vi "Stacking Test.vi"(11 "Pilot-CoPilot Gamepad Controls":T1) -> ()   [LabVIEW 2014]
uses:
  Subsystems VIs/Robot Control Outputs 2015.ctl
  <vilib>/Rock Robotics/WPI/Solenoid/WPI_SolenoidValue.ctl
  <vilib>/Rock Robotics/Network Tables/SD Write Boolean Array.vi
  Global Variables/Refnum Names.vi
  Global Variables/Sensor Data (Edited).vi
  <vilib>/Rock Robotics/Network Tables/SD Write Numeric Array.vi
  <vilib>/Rock Robotics/Network Tables/SD Write Boolean.vi
  <vilib>/Rock Robotics/WPI/Solenoid/WPI_SolenoidSetEnum.vi
panel:
  out "Motor Output":dbl
  # "CB = control board"
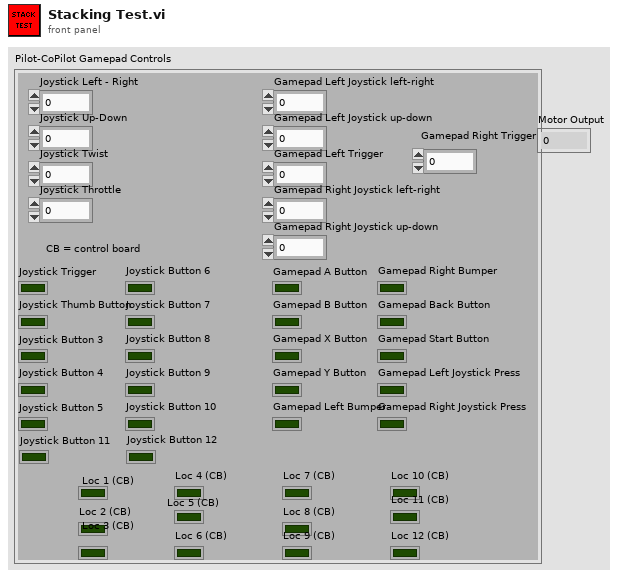
[diagram p1: front panel]
types:
  T1 = typedef "Robot Control Outputs 2015.ctl" = cluster{"Gamepad Left Joystick left-right":dbl, "Gamepad Left Joystick up-down":dbl, "Gamepad A Button":bool, "Gamepad B Button":bool, "Gamepad X Button":bool, "Gamepad Y Button":bool, "Gamepad Left Bumper":bool, "Gamepad Right Bumper":bool, "Gamepad Back Button":bool, "Gamepad Start Button":bool, "Gamepad Left Joystick Press":bool, "Gamepad Right Joystick Press":bool, "Joystick Trigger":bool, "Joystick Thumb Button":bool, "Joystick Button 3":bool, "Joystick Button 4":bool, "Joystick Button 5":bool, "Joystick Button 6":bool, "Joystick Button 7":bool, "Joystick Button 8":bool, "Joystick Button 9":bool, "Joystick Button 10":bool, "Gamepad Left Trigger":dbl, "Gamepad Right Joystick left-right":dbl, "Gamepad Right Joystick up-down":dbl, "Joystick Left - Right":dbl, "Joystick Up-Down":dbl, "Joystick Twist":dbl, "Joystick Throttle":dbl, "Loc 1 (CB)":bool, "Loc 4 (CB)":bool, "Gamepad Right Trigger":dbl, "Loc 2 (CB)":bool, "Loc 3 (CB)":bool, "Loc 5 (CB)":bool, "Loc 6 (CB)":bool, "Loc 7 (CB)":bool, "Loc 10 (CB)":bool, "Loc 8 (CB)":bool, "Loc 9 (CB)":bool, "Loc 11 (CB)":bool, "Loc 12 (CB)":bool, "Joystick Button 11":bool, "Joystick Button 12":bool}
  T2 = typedef "WPI_SolenoidValue.ctl" = enum16{"Off", "On", "Forward", "Reverse"}
  T3 = typedef "WPI_SolenoidDevRef.ctl" = cluster{"DevStatus":errorcluster, "Pneumatics Control Module":u8, "Forward Solenoid Channel":T4, "Reverse Solenoid Channel":T4}
  T4 = typedef "WPI_SolenoidChannel.ctl" = enum8{"Solenoid 0", "Solenoid 1", "Solenoid 2", "Solenoid 3", "Solenoid 4", "Solenoid 5", "Solenoid 6", "Solenoid 7", "Invalid"}
  T5 = typedef "WPI_MotorControlDeviceRef.ctl" = cluster{"DeviceStatus":errorcluster, "Type":T6, "PWM":cluster{"Controller":T7, "PWM Channel":T8, "DeadBand":T9}, "CAN":cluster{"Device Number":u8, "Control Mode":T10, "Semaphore":T11, "Max Vout":dbl, "TalonSRX Control Mode":T12}, "Invert":bool, "TransformRef":T13, "InvTransformRef":T13}
  T6 = typedef "WPI_MotorControlType.ctl" = enum16{"PWM", "CAN", "CANTalonSRX"}
  T7 = typedef "FPGA_TypedefDigitalModule.ctl" = enum16{"Controller 1"}
  T8 = typedef "FPGA_DIOPWMChannel.ctl" = enum8{"PWM 0", "PWM 1", "PWM 2", "PWM 3", "PWM 4", "PWM 5", "PWM 6", "PWM 7", "PWM 8", "PWM 9", "PWM MXP 0", "PWM MXP 1", "PWM MXP 2", "PWM MXP 3", "PWM MXP 4", "PWM MXP 5", "PWM MXP 6", "PWM MXP 7", "PWM MXP 8", "PWM MXP 9", "Invalid"}
  T9 = typedef "WPI_PWMDeadband.ctl" = cluster{"Name":string, "maxPositivePwm":i32, "minPositivePwm":i32, "centerPwm":i32, "maxNegativePwm":i32, "minNegativePwm":i32, "angularRange":u16}
  T10 = typedef "WPI_CANJaguar_ControlMode.ctl" = enum8{"Percent VBus", "Current", "Speed", "Position", "Voltage"}
  T11 = typedef "Semaphore RefNum" = refnum<k1>
  T12 = typedef "WPI_CANTalonSRX_APIControlMode.ctl" = enum8{"Percent VBus", "Speed", "Position", "Slave", "Unchanged / Invalid"}
  T13 = typedef "WPI_PWMTransform_ConPane.ctl" = refnum<vi>
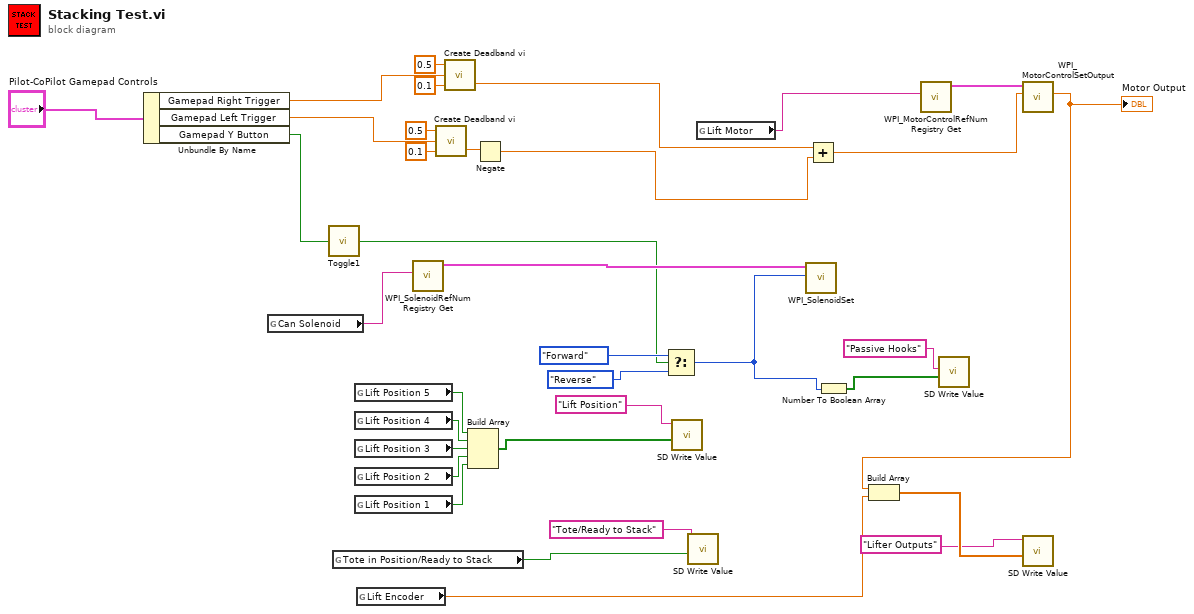
[diagram p0: block diagram]
diagram:
  n1 = Unbundle By Name("Pilot-CoPilot Gamepad Controls") -> ("Gamepad Right Trigger"=w9:dbl, "Gamepad Left Trigger"=w4:dbl, "Gamepad Y Button"=w34:bool)
  n2 = global read "Refnum Names.vi" "Can Solenoid"() -> (w13:string)
  n3 = call "Toggle1.vi"("Boolean"=w34) -> ("Driver Switch 2"=w14:bool)
  n4 = global read "Sensor Data (Edited).vi" "Tote in Position/Ready to Stack"() -> (w19:bool)
  n5 = global read "Sensor Data (Edited).vi" "Lift Position 5"() -> (w33:bool)
  n6 = global read "Sensor Data (Edited).vi" "Lift Position 4"() -> (w32:bool)
  n7 = global read "Sensor Data (Edited).vi" "Lift Position 3"() -> (w31:bool)
  n8 = global read "Sensor Data (Edited).vi" "Lift Position 2"() -> (w30:bool)
  n9 = global read "Sensor Data (Edited).vi" "Lift Position 1"() -> (w29:bool)
  n10 = global read "Sensor Data (Edited).vi" "Lift Encoder"() -> (w24:dbl)
  n11 = call <vilib>:"WPI_SolenoidRefNum Registry Get.vi"("refnum name"=w13) -> ("SolenoidDevRef"=w17:T3)  [unwired: 9 in, 1 out]
  n12 = call "Create Deadband vi.vi"("Input Deadband"=0.1, "Input"=w4, "Output Upper Limit"=0.5) -> ("Output"=w3:dbl)  [unwired: 1 in]
  n13 = call "Create Deadband vi.vi"("Input Deadband"=0.1, "Input"=w9, "Output Upper Limit"=0.5) -> ("Output"=w1:dbl)  [unwired: 1 in]
  n14 = Build Array(w33, w32, w31, w30, w29) -> (w28:bool[])
  n15 = Negate(x=w3) -> (-x=w2:dbl)
  n16 = Select(t=WPI_SolenoidValue."Forward" ("Value"), s=w14, f=WPI_SolenoidValue."Reverse" ("Value")) -> (s? t:f=w12:T2)
  n17 = call-poly <vilib>:"SD Write Value.vi"("Boolean Array"=w28, "Name"="Lift Position") -> ()  [unwired: 8 in, 2 out]
  n18 = call-poly <vilib>:"SD Write Value.vi"("Boolean"=w19, "Name"="Tote/Ready to Stack") -> ()  [unwired: 8 in, 2 out]
  n19 = global read "Refnum Names.vi" "Lift Motor"() -> (w25:string)
  n20 = call-poly <vilib>:"WPI_SolenoidSet.vi"("Value"=w12, "SolenoidDevRef"=w17) -> ()  [unwired: 8 in, 2 out]
  n21 = Add(x=w1, y=w2) -> (x+y=w18:dbl)
  n22 = Number To Boolean Array(number=w12) -> (Boolean array=w11:bool[])
  n23 = call <vilib>:"WPI_MotorControlRefNum Registry Get.vi"("refnum name"=w25) -> ("MotorControlDevRef"=w26:T5)  [unwired: 9 in, 1 out]
  n24 = call-poly <vilib>:"SD Write Value.vi"("Boolean Array"=w11, "Table Prefix"="Passive Hooks" ("Name")) -> ()  [unwired: 8 in, 2 out]
  n25 = call <vilib>:"WPI_MotorControlSetOutput.vi"("Output"=w18, "MotorControlDevRef"=w26) -> ("Motor Output"=w23:dbl)  [unwired: 7 in, 2 out]
  "Motor Output" <- w23
  n26 = Build Array(w23, w24) -> (w22:dbl[])
  n27 = call-poly <vilib>:"SD Write Value.vi"("Numeric Array"=w22, "Name"="Lifter Outputs") -> ()  [unwired: 8 in, 2 out]
